vi "Intialize EtherCAT youBot Arm.vi"(8 "error in (no error)":errorcluster, 11 "arm slave infos":T1[](array[typedef]) {"nodeAddr" format="%.0x"}) -> (0 "error out":errorcluster, 3 "KUKA youBot arm_EtherCAT out":refnum<class "NI_Robotics_KUKA youBot Arm_EtherCAT.lvclass">)   [LabVIEW 2017, in "NI_Robotics_KUKA youBot Host.lvlib" / "NI_Robotics_KUKA youBot Arm_EtherCAT.lvclass"]
uses:
  <vilib>/robotics/KUKA youBot/Basic Device/Arm EtherCAT/NI_Robotics_KUKA youBot Arm_EtherCAT.lvclass
  c:/Program Files (x86)/National Instruments/LabVIEW 2017/vi.lib/robotics/Kinematics/Robot/NI_Robotics_Serial Robot Arm.lvclass
  c:/Program Files (x86)/National Instruments/LabVIEW 2017/vi.lib/robotics/KUKA youBot/Basic Device/Arm/NI_Robotics_KUKA youBot Arm.lvclass
  <vilib>/robotics/KUKA youBot/EtherCAT/Motor Slave Info.ctl
  <vilib>/robotics/KUKA youBot/EtherCAT/LowLevel/Mater Handler.ctl
  <vilib>/robotics/KUKA youBot/Motor/Arm Motor EtherCAT/Arm Motor Parameter.ctl
  <vilib>/robotics/Kinematics/DH Dynamic Parameters.ctl
  <vilib>/Analysis/Matrix/Datatypes/RealMatrix.ctl
  <vilib>/robotics/KUKA youBot/Motor/Arm Motor EtherCAT/NI_Robotics_KUKA youBot Arm Motor_EtherCAT.lvclass
  c:/Program Files (x86)/National Instruments/LabVIEW 2017/vi.lib/robotics/KUKA youBot/Motor/Arm Motor/NI_Robotics_KUKA youBot Arm Motor.lvclass
  <vilib>/robotics/KUKA youBot/Basic Device/Gripper EtherCAT/NI_Robotics_KUKA youBot Gripper_EtherCAT.lvclass
  c:/Program Files (x86)/National Instruments/LabVIEW 2017/vi.lib/robotics/KUKA youBot/Basic Device/Gripper/NI_Robotics_KUKA youBot Gripper.lvclass
  <vilib>/Analysis/7linalg.llb/Create Special Real Matrix.vi
  <vilib>/robotics/KUKA youBot/Basic Device/Arm/NI_Robotics_KUKA youBot Arm.lvclass
  <vilib>/robotics/Kinematics/Robot/NI_Robotics_Serial Robot Arm.lvclass
  <vilib>/robotics/Kinematics/NI_Kinematics.lvlib
  <vilib>/Analysis/NI_AALPro.lvlib
  <vilib>/robotics/Utilities/NI_Robotics Utilities.lvlib
  <vilib>/Analysis/Matrix/NI_Matrix.lvlib
  <vilib>/robotics/Kinematics/Link/NI_Robotics_Link.lvclass
  <vilib>/robotics/KUKA youBot/NI_Robotics_KUKA youBot Host.lvlib
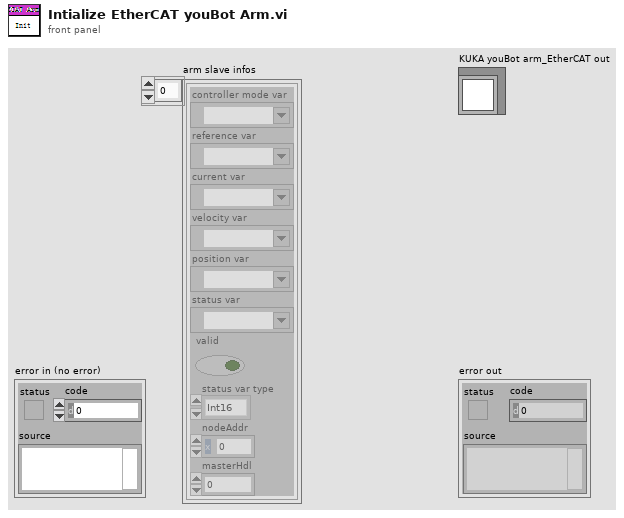
[diagram p1: front panel]
types:
  T1 = typedef "NI_Robotics_KUKA youBot Host.lvlib/Motor Slave Info.ctl" = cluster{"controller mode var":refnum<k21>, "reference var":refnum<k21>, "current var":refnum<k21>, "velocity var":refnum<k21>, "position var":refnum<k21>, "status var":refnum<k21>, "valid":bool, "status var type":enum16{"Int16", "Int32"}, "nodeAddr":u16, "masterHdl":T2}
  T2 = typedef "NI_Robotics_KUKA youBot Host.lvlib/Mater Handler.ctl" = i32
  T3 = typedef "NI_Robotics_KUKA youBot Host.lvlib/NI_Robotics_KUKA youBot Arm Motor_EtherCAT.lvclass/Arm Motor Parameter.ctl" = cluster{"ticks per radian":dbl, "ticks offset":i32, "calibration max current (A)":dbl, "torqure constant (Nm/A)":dbl, "do calibration?":bool, "positive calibtration direction?":bool}
  T4 = typedef "DH Dynamic Parameters.ctl" = cluster{"mass":dbl, "gear ratio":dbl, "motor inertia":dbl, "center of gravity":dbl[], "viscous friction":dbl, "positive coulomb friction":dbl, "negative coulomb friction":dbl, "inertia matrix":T5}
  T5 = typedef "NI_Matrix.lvlib/RealMatrix.ctl" = dbl[][]
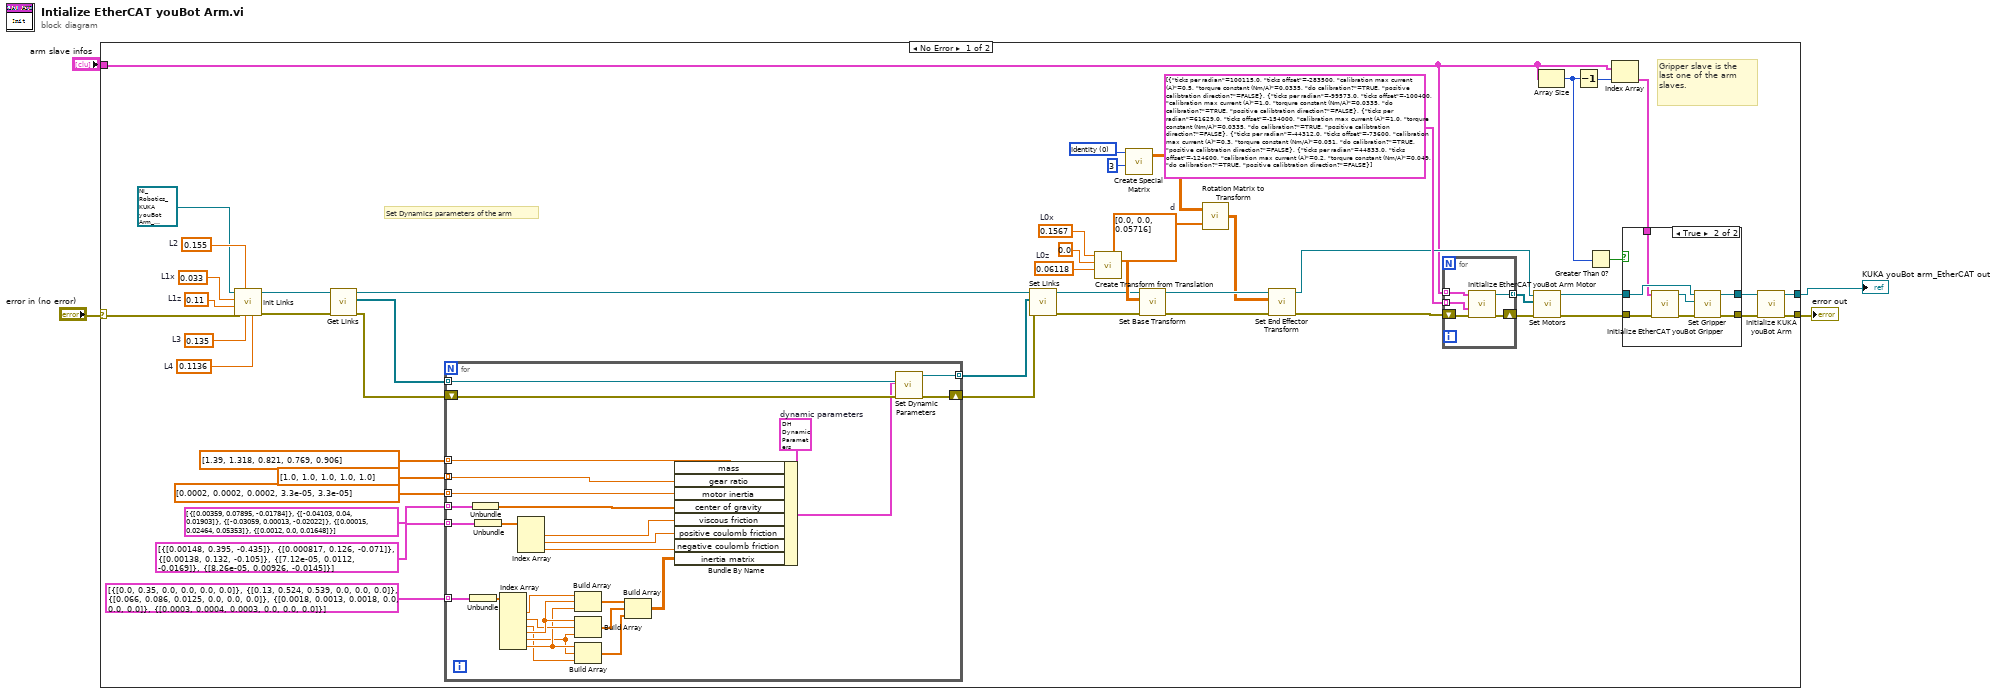
[diagram p0: block diagram]
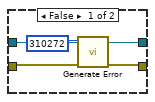
[diagram p2: hidden frame]
diagram:
  n1 = case shown="No Error" "error in (no error)" {
    selector: "error in (no error)" -> [w30 w98]
    tunnel: [w50 w98] -> w3
    tunnel: [w51 _] -> w2
    tunnel: "arm slave infos" -> [w25 _]
    frame No Error {
      w20 = 0.1136  # L4
      w33 = 0 items=["Identity", "Diagonal", "Toeplitz", "Vandermonde", "Companion", "Hankel", "Hadamard", "Wilkinson", "Hilbert", "Inverse Hilbert", "Rosser", "Pascal"] ("matrix type")
      w38 = dbl[] [0.0, 0.0, 0.05716]  # d
      w34 = 0.135  # L3
      w35 = 0.155  # L2
      w36 = 0.11  # L1z
      w37 = 0.033  # L1x
      w42 = 0.06118  # L0z
      w44 = 0.1567  # L0x
      # "Set Dynamics parameters of the arm"
      # "Gripper slave is the last one of the arm slaves."
      n2 = call-dynamic "Init Links.vi"("L4"=w20, "L3"=w34, "L2"=w35, "error in (no error)"=w30, "L1z"=w36, "L1x"=w37, "NI_Robotics_5R Type 1 Serial Arm Class in"=refnum<class "NI_Robotics_KUKA youBot Arm_EtherCAT.lvclass"> refnum ("NI_Robotics_KUKA youBot Host.lvlib:NI_Robotics_KUKA youBot Arm_EtherCAT.lvclass")) -> ("error out"=w12:errorcluster, "NI_Robotics_5R Type 1 Serial Arm Class out"=w13:refnum<class "NI_Robotics_KUKA youBot Arm_EtherCAT.lvclass">)  [unwired: 3 in]
      n3 = call <vilib>:"Get Links.vi"("error in (no error)"=w12, "serial arm in"=w13) -> ("error out"=w11:errorcluster, "links"=w10:refnum<class "NI_Robotics_Link.lvclass">[], "serial arm out"=w5:refnum<class "NI_Robotics_KUKA youBot Arm_EtherCAT.lvclass">)  [unwired: 7 in]
      n4 = for {
        tunnel: w10 -> [w58] mode=indexing
        tunnel: dbl[] [1.39, 1.318, 0.821, 0.769, 0.906] -> [w80] mode=indexing
        tunnel: dbl[] [1.0, 1.0, 1.0, 1.0, 1.0] -> [w79] mode=indexing
        tunnel: dbl[] [0.0002, 0.0002, 0.0002, 3.3e-05, 3.3e-05] -> [w78] mode=indexing
        tunnel: cluster{dbl[]}[] [{[0.00359, 0.07895, -0.01784]}, {[-0.04103, 0.04, 0.01903]}, {[-0.03059, 0.00013, -0.02022]}, {[0.00015, 0.02464, 0.05353]}, {[0.0012, 0.0, 0.01648]}] -> [w77] mode=indexing
        tunnel: cluster{dbl[]}[] [{[0.00148, 0.395, -0.435]}, {[0.000817, 0.126, -0.071]}, {[0.00138, 0.132, -0.105]}, {[7.12e-05, 0.0112, -0.0169]}, {[8.26e-05, 0.00926, -0.0145]}] -> [w75] mode=indexing
        tunnel: cluster{dbl[]}[] [{[0.0, 0.35, 0.0, 0.0, 0.0, 0.0]}, {[0.13, 0.524, 0.539, 0.0, 0.0, 0.0]}, {[0.066, 0.086, 0.0125, 0.0, 0.0, 0.0]}, {[0.0018, 0.0013, 0.0018, 0.0, 0.0, 0.0]}, {[0.0003, 0.0004, 0.0003, 0.0, 0.0, 0.0]}] -> [w61] mode=indexing
        tunnel: [w55] -> w7 mode=indexing
        shift-right: [w54] -> w6
        shift-left: w11 -> [w57]
        w81 = T4 {"mass"=0.0, "gear ratio"=0.0, "motor inertia"=0.0, "center of gravity"=[], "viscous friction"=0.0, "positive coulomb friction"=0.0, "negative coulomb friction"=0.0, "inertia matrix"=[[0.0, 0.0, 0.0], [0.0, 0.0, 0.0], [0.0, 0.0, 0.0]]}  # dynamic parameters
        n5 = Unbundle(w61) -> (w60:dbl[])
        n6 = Unbundle(w77) -> (w76:dbl[])
        n7 = Unbundle(w75) -> (w74:dbl[])
        n8 = Index Array(array=w60) -> (element #1=w70:dbl, element #2=w68:dbl, element #3=w65:dbl, element #4=w69:dbl, element #5=w66:dbl, element #6=w67:dbl)  [unwired: 6 in]
        n9 = Index Array(array=w74) -> (element #1=w73:dbl, element #2=w72:dbl, element #3=w71:dbl)  [unwired: 3 in]
        n10 = Build Array(w70, w69, w67) -> (w64:dbl[])
        n11 = Build Array(w69, w68, w66) -> (w63:dbl[])
        n12 = Build Array(w67, w66, w65) -> (w62:dbl[])
        n13 = Build Array(w64, w63, w62) -> (w59:dbl[][])
        n14 = Bundle By Name(cluster=w81, "mass"=w80, "gear ratio"=w79, "motor inertia"=w78, "center of gravity"=w76, "viscous friction"=w73, "positive coulomb friction"=w72, "negative coulomb friction"=w71, "inertia matrix"=w59) -> (w56:T4)
        n15 = call <vilib>:"Set Dynamic Parameters.vi"("error in (no error)"=w57, "dynamic parameters"=w56, "link in"=w58) -> ("error out"=w54:errorcluster, "link out"=w55:refnum<class "NI_Robotics_Link.lvclass">)  [unwired: 7 in]
      }
      n16 = call <vilib>:"Set Links.vi"("error in (no error)"=w6, "links"=w7, "serial arm in"=w5) -> ("error out"=w8:errorcluster, "serial arm out"=w9:refnum<class "NI_Robotics_KUKA youBot Arm_EtherCAT.lvclass">)  [unwired: 7 out]
      n17 = call <vilib>:"Create Transform from Translation.vi"("z"=w42, "y"=0.0, "x"=w44) -> ("transform"=w45:T5)  [unwired: 8 in]
      n18 = call-poly <vilib>:"Create Special Matrix.vi"("matrix type"=w33, "matrix size"=3) -> ("Special Matrix"=w31:T5)  [unwired: 3 in, 1 out]
      n19 = call <vilib>:"Set Base Transform.vi"("error in (no error)"=w8, "base transform"=w45, "serial arm in"=w9) -> ("error out"=w41:errorcluster, "serial arm out"=w40:refnum<class "NI_Robotics_KUKA youBot Arm_EtherCAT.lvclass">)  [unwired: 7 in]
      n20 = call <vilib>:"Rotation Matrix to Transform.vi"("translation vector"=w38, "rotation matrix"=w31) -> ("transform"=w39:T5)
      n21 = call <vilib>:"Set End Effector Transform.vi"("error in (no error)"=w41, "end effector transform"=w39, "serial arm in"=w40) -> ("error out"=w28:errorcluster, "serial arm out"=w27:refnum<class "NI_Robotics_KUKA youBot Arm_EtherCAT.lvclass">)  [unwired: 7 in]
      n22 = for {
        shift-right: [w97] -> w53
        shift-left: w28 -> [w95]
        tunnel: [w96] -> w52 mode=indexing
        tunnel: w25 -> [w93] mode=indexing
        tunnel: T3[] [{"ticks per radian"=100115.0, "ticks offset"=-283500, "calibration max current (A)"=0.5, "torqure constant (Nm/A)"=0.0335, "do calibration?"=TRUE, "positive calibtration direction?"=FALSE}, {"ticks per radian"=-99573.0, "ticks offset"=-100400, "calibration max current (A)"=1.0, "torqure constant (Nm/A)"=0.0335, "do calibration?"=TRUE, "positive calibtration direction?"=FALSE}, {"ticks per radian"=61629.0, "ticks offset"=-154000, "calibration max current (A)"=1.0, "torqure constant (Nm/A)"=0.0335, "do calibration?"=TRUE, "positive calibtration direction?"=FALSE}, {"ticks per radian"=-44312.0, "ticks offset"=-73600, "calibration max current (A)"=0.3, "torqure constant (Nm/A)"=0.051, "do calibration?"=TRUE, "positive calibtration direction?"=FALSE}, {"ticks per radian"=44833.0, "ticks offset"=-124600, "calibration max current (A)"=0.2, "torqure constant (Nm/A)"=0.049, "do calibration?"=TRUE, "positive calibtration direction?"=FALSE}] -> [w94] mode=indexing
        n23 = call <vilib>:"Initialize EtherCAT youBot Arm Motor.vi"("error in (no error)"=w95, "arm motor param"=w94, "motor slave info in"=w93) -> ("error out"=w97:errorcluster, "KUKA youBot arm motor_EtherCAT out"=w96:refnum<class "NI_Robotics_KUKA youBot Arm Motor_EtherCAT.lvclass">)  [unwired: 7 in]
      }
      n24 = call <vilib>:"Set Motors.vi"("error in (no error)"=w53, "motors"=w52, "KUKA youBot arm in"=w27) -> ("error out"=w48:errorcluster, "KUKA youBot arm out"=w47:refnum<class "NI_Robotics_KUKA youBot Arm_EtherCAT.lvclass">)  [unwired: 7 in]
      n25 = Array Size(array=w25) -> (size(s)=w22:i32)
      n26 = Decrement(x=w22) -> (x-1=w26:i32)
      n27 = Greater Than 0?(x=w22) -> (x > 0?=w21:bool)
      n28 = Index Array(array=w25, index=w26) -> (element=w24:T1)
      n29 = case shown="True" w21 {
        tunnel: w48 -> [w84 w92]
        tunnel: w47 -> [w85 w91]
        tunnel: [w85 w90] -> w46
        tunnel: w24 -> [_ w87]
        tunnel: [w83 w86] -> w23
        frame False {
          n30 = call <vilib>:"Generate Error.vi"("error in (no error)"=w84, "code"=310272) -> ("error out"=w83:errorcluster)  [unwired: 9 in]
        }
        frame True {
          n31 = call <vilib>:"Initialize EtherCAT youBot Gripper.vi"("error in (no error)"=w92, "gripper slave info in"=w87) -> ("error out"=w89:errorcluster, "KUKA youBot gripper_EtherCAT out"=w88:refnum<class "NI_Robotics_KUKA youBot Gripper_EtherCAT.lvclass">)  [unwired: 8 in]
          n32 = call-dynamic "Set Gripper.vi"("error in (no error)"=w89, "KUKA youBot gripper"=w88, "KUKA youBot arm in"=w91) -> ("error out"=w86:errorcluster, "KUKA youBot arm out"=w90:refnum<class "NI_Robotics_KUKA youBot Arm_EtherCAT.lvclass">)  [unwired: 7 in]
        }
      }
      n33 = call <vilib>:"Initialize KUKA youBot Arm.vi"("error in (no error)"=w23, "KUKA youBot arm in"=w46) -> ("error out"=w50:errorcluster, "KUKA youBot arm out"=w51:refnum<class "NI_Robotics_KUKA youBot Arm_EtherCAT.lvclass">)  [unwired: 8 in]
    }
    frame Error {
    }
  }
  "error out" <- w3
  "KUKA youBot arm_EtherCAT out" <- w2
